vi "EnqueueError.vi"(8 "ErrorArray In":errorcluster[](array[cluster])) -> (0 "ErrorArray Out":errorcluster[](array[cluster]))   [LabVIEW 2014, in "TestFramework.lvlib"]
uses:
  TestFramework.lvlib
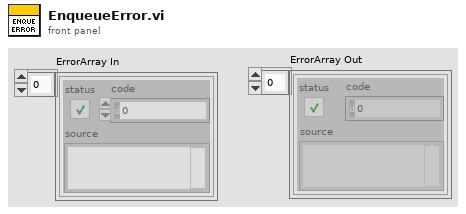
[diagram p1: front panel]
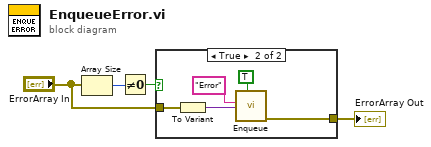
[diagram p0: block diagram]
diagram:
  n1 = Array Size(array="ErrorArray In") -> (size(s)=w4:i32)
  n2 = Not Equal To 0?(x=w4) -> (x != 0?=w3:bool)
  n3 = case shown="True" w3 {
    tunnel: "ErrorArray In" -> [_ w8]
    tunnel: [_ w5] -> w1
    frame False {
    }
    frame True {
      n4 = To Variant(anything=w8) -> (Variant=w7:variant)
      n5 = call "Enqueue.vi"("Priority (f)"=TRUE, "Data"=w7, "Msg"="Error") -> ("ErrorArray Out"=w5:errorcluster[])  [unwired: 8 in]
    }
  }
  "ErrorArray Out" <- w1
